vi "WT Control Main.vi"() -> ()   [LabVIEW 2017]
uses:
  <vilib>/Platform/TimedLoop/XDataNode/timing_clust.ctl
  <vilib>/Platform/TimedLoop/XDataNode/nitl_modes.ctl
  <vilib>/Platform/TimedLoop/XDataNode/wakeup.ctl
  <vilib>/Analysis/baseanly.llb/Mean (DBL).vi
  <vilib>/DAQmx/read.llb/DAQmx Read (Analog 1D DBL NChan 1Samp).vi
  <vilib>/DAQmx/miscellaneous.llb/DAQmx Fill In Error Info.vi
  Globals/mainWTControl.vi
  <vilib>/platform/TimedLoop/XDataNode/XDataNode.xnode
  <vilib>/Analysis/NI_AALBase.lvlib
  <vilib>/Platform/TimedLoop/XDataNode/XDNodeRunTimeDep.lvlib
panel:
  out "Boolean":bool
  in  "Blank Button":bool
  out "Fan 2 (A)":dbl
  out "Fan 1 (A)":dbl
  in  "Stop Button":bool
  out "Air Density (kg/m3)":dbl
  out "Tunnel Temp. (C)":sgl(slide) scale=0.0..20.0 scale format="%#_4g"
  in  "Fan 2 (V)":dbl
  in  "Fan 1 (V)":dbl
  in  "Fans Power Switch":bool
  out "Wind Velocity":dbl format="%#_4g"
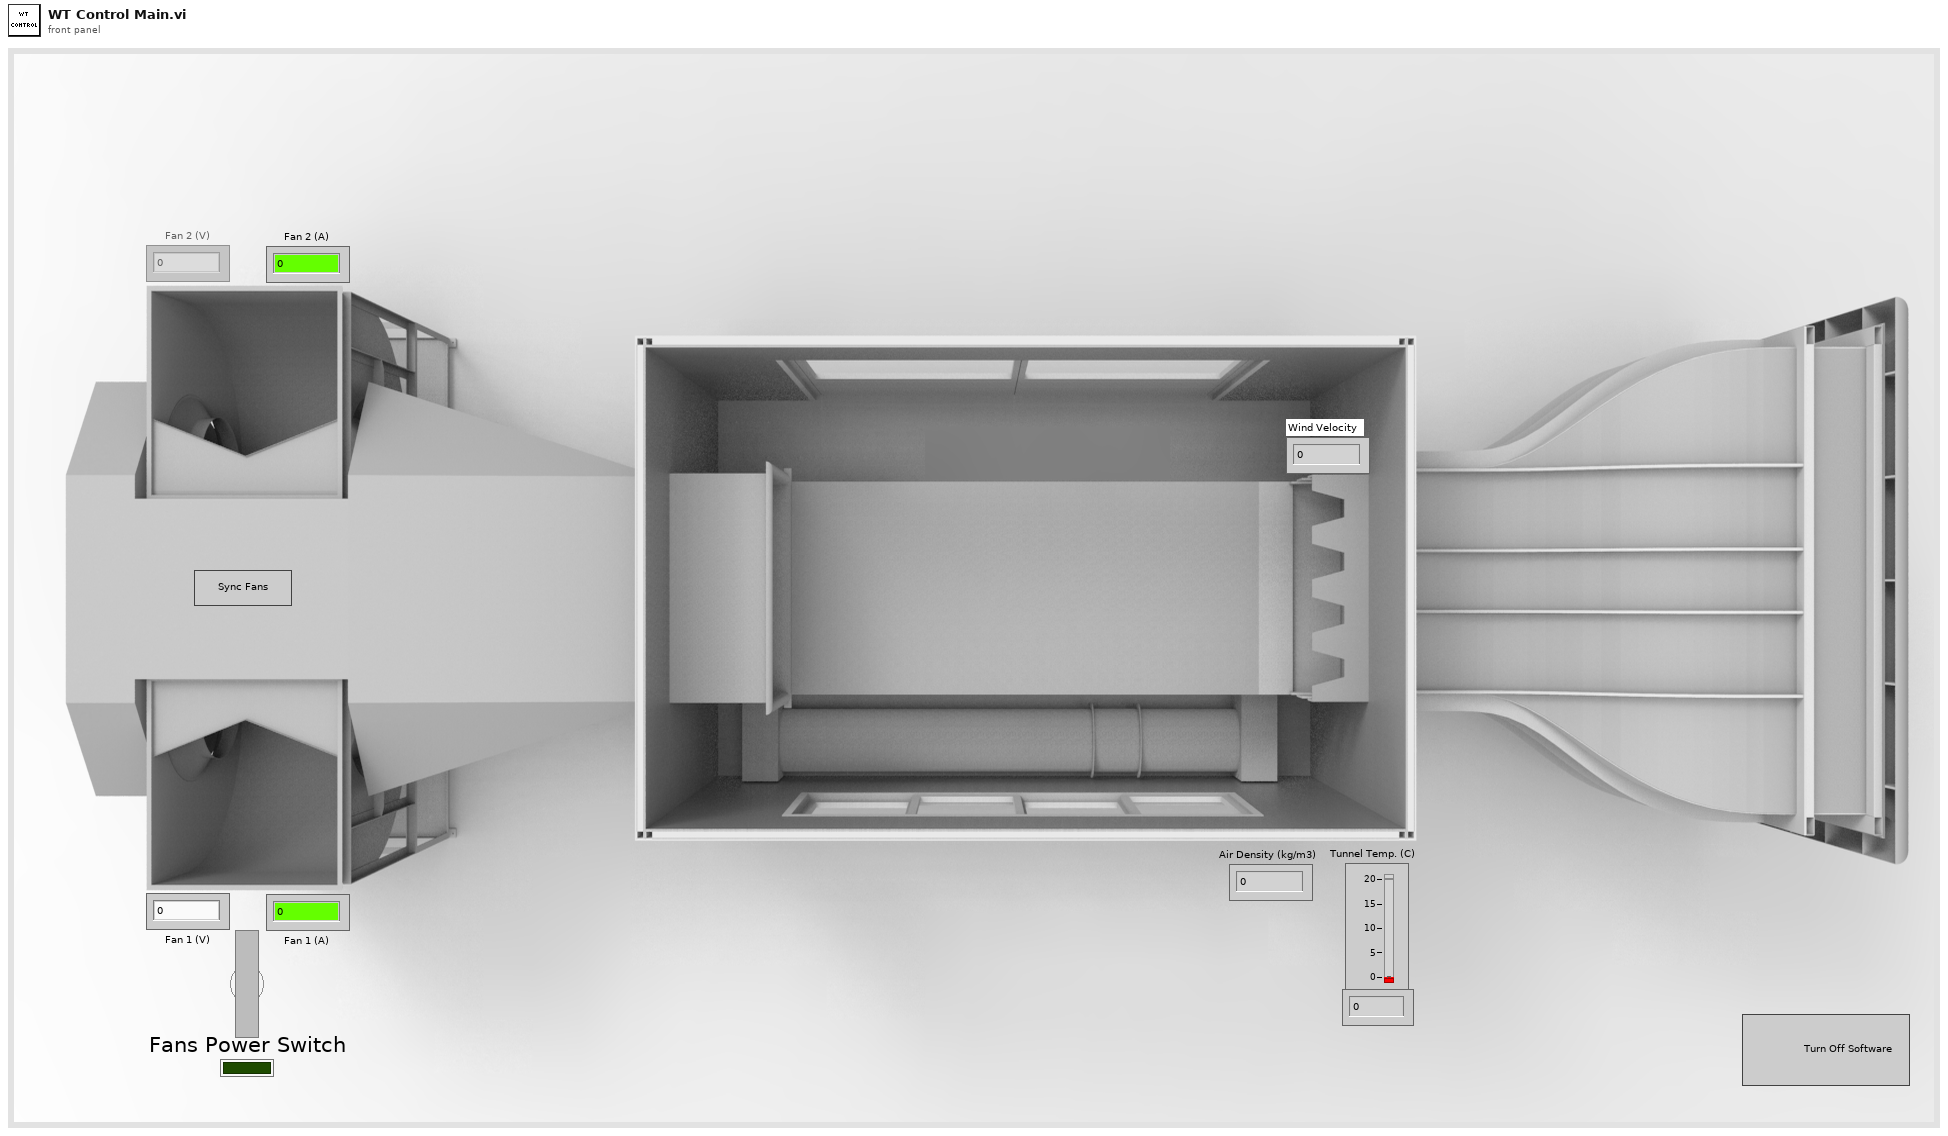
[diagram p1: front panel]
types:
  T1 = enum8{"Enabled", "Disabled", "Disabled and Grayed Out"}
  T2 = typedef "XDNodeRunTimeDep.lvlib/timing_clust.ctl" = cluster{"Expected End [f-1]":u64, "Actual End [f-1]":u64, "Finished Late? [f-1]":bool, "Expected End [i-1]":u64, "Actual End [i-1]":u64, "Finished Late? [i-1]":bool, "Expected Start [i]":u64, "Actual Start [i]":u64, "Expected Start [f]":u64, "Actual Start [f]":u64, "Source Name":string, "Structure Name":string, "Period":i64, "Deadline":i64, "Offset":i64, "Start":i64, "Priority":i32, "Timeout":i32, "Mode":T3, "Wakeup Reason":T4, "Error":errorcluster, "Source Type":string, "Secondary Source Type":string, "Global End Time":u64, "Global Start Time":u64, "Frame Duration":u64, "Iteration Duration":u64, "Assigned CPU":i32, "I/O Scan Engine Mode":u32}
  T3 = typedef "XDNodeRunTimeDep.lvlib/nitl_modes.ctl" = enum32{"No Change", "Process missed periods, maintain original phase", "Discard missed periods, maintain original phase", "Process missed periods, ignore original phase", "Discard missed periods, ignore original phase"}
  T4 = typedef "XDNodeRunTimeDep.lvlib/wakeup.ctl" = enum32{"Normal", "Aborted", "Asynchronous wakeup", "Timing source error", "Timed loop error", "Timeout"}
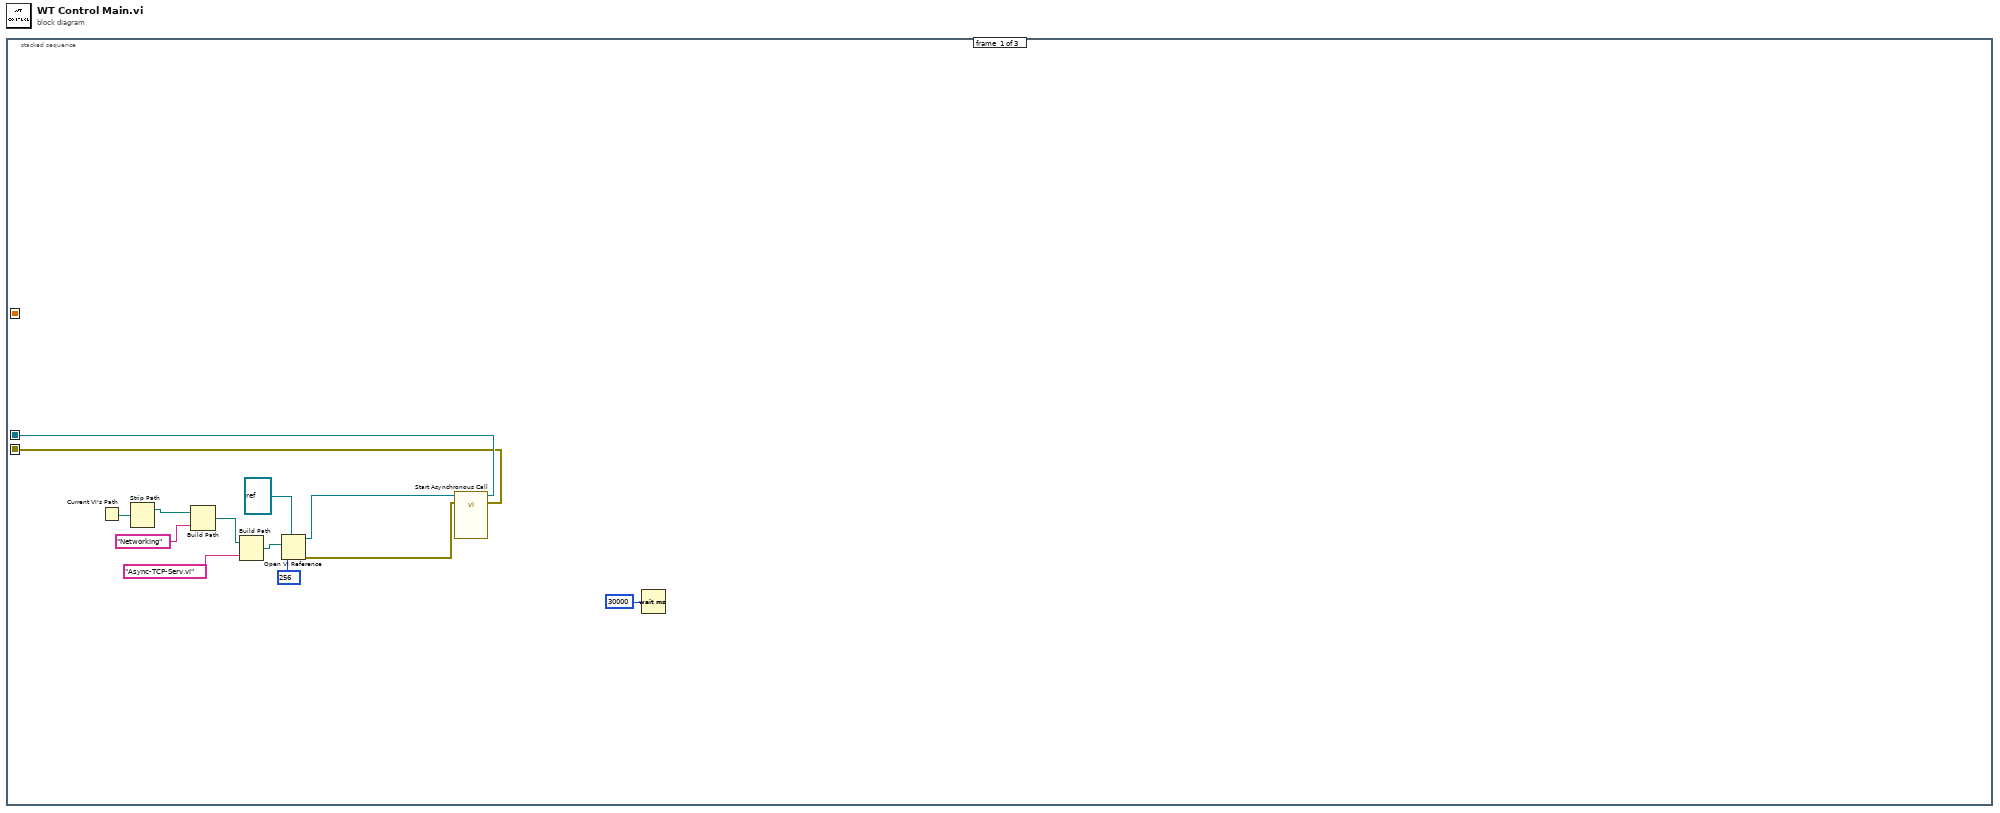
[diagram p0: block diagram]
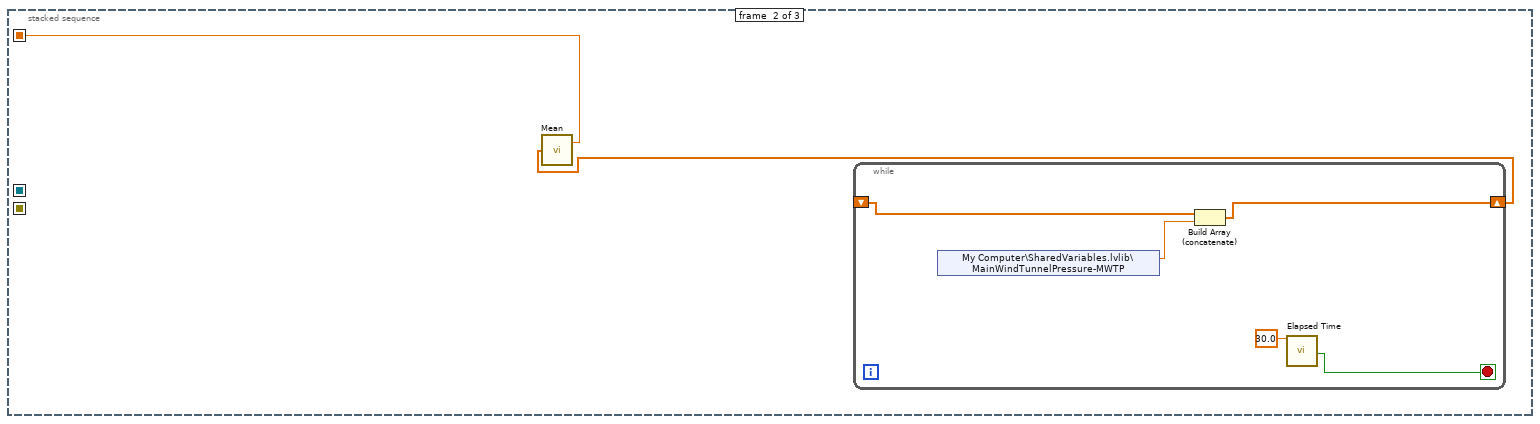
[diagram p2: hidden frame]
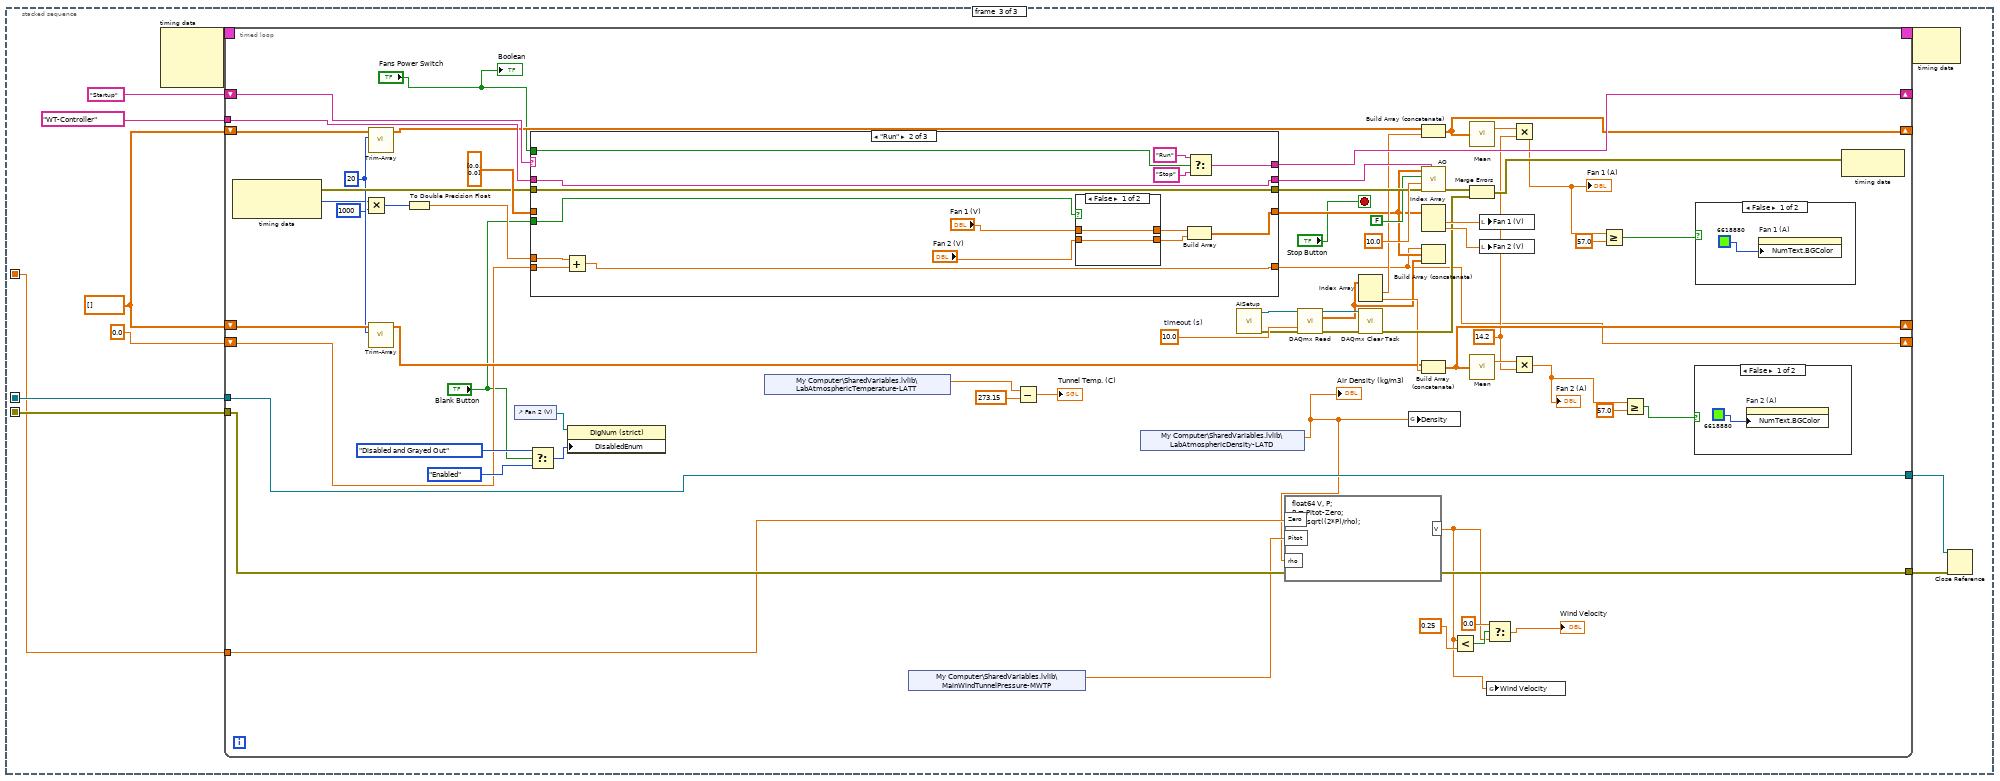
[diagram p3: hidden frame]
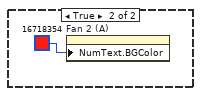
[diagram p4: hidden frame]
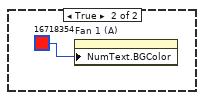
[diagram p5: hidden frame]
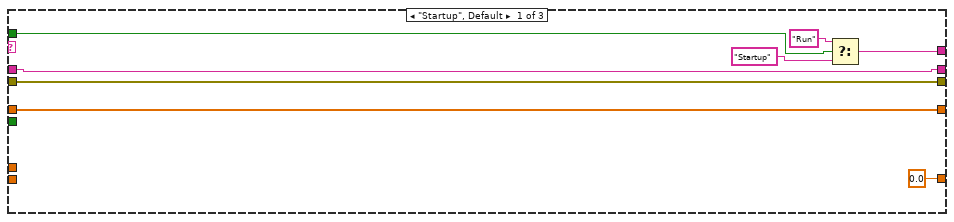
[diagram p6: hidden frame]
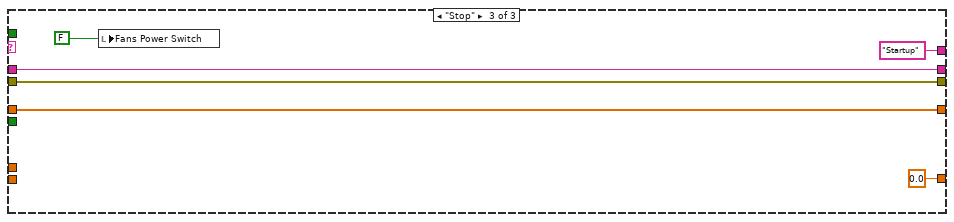
[diagram p8: hidden frame]
diagram:
  n1 = stacked-sequence {
    seq-local: [w3 _ _] -> [_ _ w25]
    seq-local: [w2 _ _] -> [_ _ w24]
    seq-local: [_ w14 _] -> [_ _ w21]
    frame #0 {
      n2 = Current VI's Path() -> (path=w13:path)
      n3 = Strip Path(path=w13) -> (stripped path=w9:path)  [unwired: 1 out]
      n4 = Build Path(base path=w9, name or relative path="Networking") -> (appended path=w8:path)
      n5 = Build Path(base path=w8, name or relative path="Async-TCP-Serv.vi") -> (appended path=w11:path)
      n6 = Open VI Reference(type specifier VI Refnum (for type only)=refnum<vi> refnum, vi path=w11, options=256) -> (vi reference=w5:refnum<vi>, error out=w4:errorcluster)  [unwired: 3 in]
      n7 = call-by-ref "Start Asynchronous Call"(reference=w5, error in=w4) -> (reference out=w3:refnum<vi>, error out=w2:errorcluster)  [unwired: 12 in]
      n8 = Wait (ms)(milliseconds to wait=u32 30000) -> ()  [unwired: 1 out]
    }
    frame #1 {
      n9 = while {
        shift-right: [w18] -> w15
        shift-left: _ -> [w17]
        stop <- w20 stop-if-true
        n10 = shared-variable "My Computer\\SharedVariables.lvlib\\MainWindTunnelPressure-MWTP"() -> (w19:dbl)  [unwired: 1 in, 1 out]
        n11 = Build Array (concatenate)(w17, w19) -> (w18:dbl[])
        n12 = call "Elapsed Time"("Time Target (s)"=30.0) -> ("Time has Elapsed"=w20:bool)  [unwired: 11 in, 7 out]
      }
      n13 = call-poly <vilib>:"Mean.vi"("X"=w15) -> ("mean"=w14:dbl)  [unwired: 1 out]
    }
    frame #2 {
      w27 = dbl[] []
      n14 = node-c288() -> (w31:T2)  [unwired: 3 in]
      n15 = timed-loop {
        shift-right: [w95] -> _
        shift-left: "Startup" -> [w96]
        tunnel: tag "WT-Controller" ("device name") -> [w94]
        timing: w31 -> [_]
        timing-out: [_] -> w30
        shift-right: [w71] -> _
        shift-left: w27 -> [w69]
        shift-right: [w70] -> _
        shift-left: w27 -> [w68]
        shift-right: [w55] -> _
        shift-left: 0.0 -> [w57]
        tunnel: w25 -> [w41]
        tunnel: w24 -> [w36]
        tunnel: [w41] -> w23
        tunnel: [w36] -> w22
        tunnel: w21 -> [w35]
        stop <- "Stop Button" stop-if-true
        w63 = 14.2 ("y")
        w66 = 20 ("length")
        w82 = 10.0  # timeout (s)
        n16 = node-c288() -> (w86:errorcluster, w60:i64)  [unwired: 1 in]
        n17 = Multiply(x=w60, y=i64 1000) -> (x*y=w58:i64)
        n18 = call "Trim-Array.vi"("length"=w66, "Array in"=w69) -> ("Array out"=w73:dbl[])  [unwired: 9 in]
        n19 = call "Trim-Array.vi"("length"=w66, "Array in"=w68) -> ("Array out"=w67:dbl[])  [unwired: 9 in]
        n20 = To Double Precision Float(number=w58) -> (double precision float=w56:dbl)
        n21 = control-ref of="Fan 2 (V)"() -> (w44:refnum<vi>)
        n22 = case shown="\"Run\"" w96 {
          tunnel: [w109 w129 "Startup" ("f")] -> w95
          tunnel: [w113 w125 w136] -> w62
          tunnel: w94 -> [w112 w124 w137]
          tunnel: [w114 w123 w135] -> w88
          tunnel: w86 -> [w114 w123 w135]
          tunnel: "Blank Button" -> [_ w126 _]
          tunnel: dbl[] [0.0, 0.0] ("appended array") -> [w113 _ w136]
          tunnel: [w112 w124 w137] -> w87
          tunnel: "Fans Power Switch" -> [w111 w122 _]
          tunnel: w57 -> [_ w119 _]
          tunnel: [0.0 w117 0.0] -> w55
          tunnel: w56 -> [_ w118 _]
          frame "Startup", Default {
            n23 = Select(t="Run" ("f"), s=w111, f="Startup") -> (s? t:f=w109:string)
          }
          frame "Run" {
            n24 = Add(x=w118, y=w119) -> (x+y=w117:dbl)
            n25 = case shown="False" w126 {
              tunnel: [w130 w132] -> w128
              tunnel: [w131 w132] -> w127
              tunnel: "Fan 1 (V)" -> [w131 w132]
              tunnel: "Fan 2 (V)" -> [w130 _]
              frame False {
              }
              frame True {
              }
            }
            n26 = Build Array(w127, w128) -> (w125:dbl[])
            n27 = Select(t="Run" ("f"), s=w122, f="Stop") -> (s? t:f=w129:string)
          }
          frame "Stop" {
            n28 = local write "Fans Power Switch"(FALSE ("POWER")) -> ()
          }
        }
        n29 = Select(t=T1."Disabled and Grayed Out" ("Disabled"), s="Blank Button", f=T1."Enabled") -> (s? t:f=w92:T1)
        n30 = property class="DigNum (strict)"(reference=w44, "DisabledEnum"=w92) -> ()  [unwired: 1 in, 2 out]
        n31 = shared-variable "My Computer\\SharedVariables.lvlib\\LabAtmosphericTemperature-LATT"() -> (w47:dbl)  [unwired: 1 in, 1 out]
        n32 = shared-variable "My Computer\\SharedVariables.lvlib\\MainWindTunnelPressure-MWTP"() -> (w34:dbl)  [unwired: 1 in, 1 out]
        n33 = Subtract(x=w47, y=273.15) -> (x-y=→"Tunnel Temp. (C)":dbl)
        n34 = shared-variable "My Computer\\SharedVariables.lvlib\\LabAtmosphericDensity-LATD"() -> (w33:dbl)  [unwired: 1 in, 1 out]
        "Air Density (kg/m3)" <- w33
        n35 = call "AISetup.vi"() -> ("error out"=w78:errorcluster, "task out"=w79:refnum<k21>)  [unwired: 10 in]
        n36 = formula code="float64 V, P;\nP = Pitot-Zero;\nV = sqrt((2*P)/rho);"("Zero"=w35, "Pitot"=w34, "rho"=w33) -> ("V"=w32:dbl)
        n37 = call-poly <vilib>:"DAQmx Read.vi"("task/channels in"=w79, "timeout"=w82, "error in"=w78) -> ("task out"=w80:refnum<k21>, "data"=w61:dbl[], "error out"=w81:errorcluster)  [unwired: 10 in]
        n38 = Index Array(array=w61) -> (element #1=w74:dbl, element #2=w72:dbl)  [unwired: 2 in]
        n39 = call <vilib>:"DAQmx Clear Task.vi"("task in"=w80, "error in"=w81) -> ("error out"=w77:errorcluster)  [unwired: 13 in]
        n40 = global write "mainWTControl.vi" "Density"(w33) -> ()
        n41 = Build Array (concatenate)(w73, w74) -> (w71:dbl[])
        n42 = call "AO.vi"("device name"=w87, "error in"=w88, "timeout (s)"=10.0, "stop (T)"=FALSE, "data"=w62) -> ("error out"=w76:errorcluster)  [unwired: 2 in, 1 out]
        n43 = Index Array(array=w62) -> (element #1=w85:dbl, element #2=w84:dbl)  [unwired: 2 in]
        n44 = Build Array (concatenate)(w55, w62, w61) -> ()  [unwired: 1 out]
        n45 = Build Array (concatenate)(w67, w72) -> (w70:dbl[])
        n46 = Less?(x=w32, y=0.25) -> (x < y?=w39:bool)
        n47 = call-poly <vilib>:"Mean.vi"("X"=w71) -> ("mean"=w65:dbl)  [unwired: 1 out]
        n48 = Merge Errors(w76, w77) -> (w75:errorcluster)
        n49 = call-poly <vilib>:"Mean.vi"("X"=w70) -> ("mean"=w64:dbl)  [unwired: 1 out]
        n50 = local write "Fan 1 (V)"(w85) -> ()
        n51 = local write "Fan 2 (V)"(w84) -> ()
        n52 = global write "mainWTControl.vi" "Wind Velocity"(w32) -> ()
        n53 = Select(t=0.0, s=w39, f=w32) -> (s? t:f=→"Wind Velocity":dbl)
        n54 = Multiply(x=w65, y=w63) -> (x*y=w53:dbl)
        "Fan 1 (A)" <- w53
        n55 = Multiply(x=w64, y=w63) -> (x*y=w49:dbl)
        "Fan 2 (A)" <- w49
        n56 = Greater Or Equal?(x=w53, y=57.0) -> (x >= y?=w51:bool)
        n57 = Greater Or Equal?(x=w49, y=57.0) -> (x >= y?=w48:bool)
        n58 = case shown="False" w48 {
          frame False {
            n59 = property on="Fan 2 (A)" class="DigNum (strict)"("NumText.BGColor"=u32 6618880) -> ()  [unwired: 2 in, 2 out]
          }
          frame True {
            n60 = property on="Fan 2 (A)" class="DigNum (strict)"("NumText.BGColor"=u32 16718354) -> ()  [unwired: 2 in, 2 out]
          }
        }
        n61 = case shown="False" w51 {
          frame False {
            n62 = property on="Fan 1 (A)" class="DigNum (strict)"("NumText.BGColor"=u32 6618880) -> ()  [unwired: 2 in, 2 out]
          }
          frame True {
            n63 = property on="Fan 1 (A)" class="DigNum (strict)"("NumText.BGColor"=u32 16718354) -> ()  [unwired: 2 in, 2 out]
          }
        }
        n64 = node-c288(w75) -> ()  [unwired: 1 out]
        "Boolean" <- "Fans Power Switch"
      }
      n65 = node-c288(w30) -> ()  [unwired: 1 out]
      n66 = Close Reference(reference=w23, error in (no error)=w22) -> ()  [unwired: 1 out]
    }
  }
